vi "Structure Handler.vi"() -> ()   [LabVIEW 2010] (continued)
            n13 = call-poly <vilib>:"DB Tools Open Connection.vi"("connection information"=w16) -> ("error out"=w19:errorcluster, "connection reference"=w26:T17)  [unwired: 7 in]
            n14 = call-poly <vilib>:"DB Tools Execute Query.vi"("error in (no error)"=w19, "SQL query"="SELECT Structure_Summary.Structure_ID, Structure_Summary.Structure_Name, Structure_Summary.Num_Atoms, DFT_Summary.Folder, DFT_Summary.Parent_Folder, DFT_Summary.[Calculation_Time_(Hrs)], OSZICAR_Summary.[Final_Energy_(eV)]\nFROM (DFT_Summary RIGHT JOIN Structure_Summary ON DFT_Summary.CONTCAR_Structure_ID = Structure_Summary.Structure_ID) LEFT JOIN OSZICAR_Summary ON DFT_Summary.OSZICAR_ID = OSZICAR_Summary.OSZICAR_ID\nORDER BY  DFT_Summary.Parent_Folder, Structure_Summary.Structure_Name;", "connection reference"=w26) -> ("error out"=w21:errorcluster, "recordset reference"=w23:T18)  [unwired: 5 in]
            n15 = call "Column Headers from SQL Query Recordset.vi"("error in (no error)"=w21, "recordset reference"=w23) -> ("error out"=w20:errorcluster, "columns"=w14:string[], "Recordset reference Out"=w22:T18)  [unwired: 6 in, 1 out]
            n16 = call-poly <vilib>:"DB Tools Fetch Recordset Data.vi"("error in (no error)"=w20, "recordset reference"=w22) -> ("error out"=w24:errorcluster, "recordset data"=w18:variant[][], "recordset reference out"=w25:T18)  [unwired: 3 in]
            n17 = for {
              tunnel: w18 -> [w30] mode=indexing
              tunnel: [w29] -> w17 mode=indexing
              n18 = for {
                tunnel: w30 -> [w33] mode=indexing
                tunnel: [w31] -> w29 mode=indexing
                n19 = xnode "Database Variant To Data"("database variant"=w33, "type"="") -> ("data"=w31:string)  [unwired: 1 in, 1 out]
              }
            }
            n20 = call-poly <vilib>:"DB Tools Free Object.vi"("error in (no error)"=w24, "recordset reference"=w25) -> ("error out"=w28:errorcluster, "connection reference"=w27:T17)  [unwired: 8 in]
            n21 = call <vilib>:"DB Tools Close Connection.vi"("error in (no error)"=w28, "connection reference"=w27) -> ()  [unwired: 5 in, 1 out]
            n22 = property on="2nd search column name" class="CmbBox"("Strings[]"=w14) -> ()  [unwired: 2 in, 2 out]
            n23 = property on="Database Entries" class="MCListbox (strict)"("ColHdrString"=w14, "ItemNames"=w17) -> ()  [unwired: 2 in, 2 out]
            n24 = property on="1st search column name" class="CmbBox"("Strings[]"=w14) -> ()  [unwired: 2 in, 2 out]
          }
          frame Default {
          }
          frame "VASP" {
            n25 = property on="INCAR Defaults" class="LstBox (strict)"("Val(Sgnl)"=0 ("Value (Signaling)")) -> (error out=w66:errorcluster)  [unwired: 2 in, 1 out]
            n26 = property on="K-Points Tab" class="TabCtl (strict)"(error in=w66, "Val(Sgnl)"=enum32{"Automatic", "Manual"}."Automatic" ("K-Points Tab")) -> ()  [unwired: 1 in, 2 out]
          }
        }
      }
      event "Input Structure File": Value Change {
        n27 = event-data() -> ()  [unwired: 1 in, 5 out]
        n28 = call <vilib>:"Get File Extension.vi"("file"="Input Structure File") -> ("lowercase file extension"=w83:string)  [unwired: 7 in, 3 out]
        n29 = Strip Path(path="Input Structure File") -> (stripped path=w80:path)  [unwired: 1 out]
        n30 = case shown="\"out\"" w83 {
          tunnel: "Input Structure File" -> [w93 w95 w97 _]
          tunnel: [w92 w94 w96 _] -> w75
          frame "CONTCAR", "POSCAR", Default {
            n31 = call "Parse POSCAR.vi"("POSCAR File"=w93) -> ("Structure"=w92:T3)  [unwired: 7 in, 3 out]
          }
          frame "cif" {
            n32 = call "Parse CIF File from ATK.vi"("CIF File from ATK"=w95) -> ("Atomic Structure"=w94:T3)  [unwired: 10 in]
          }
          frame "out" {
            n33 = call "Parse GULP Output file.vi"("GULP output file"=w97) -> ("Final Structure"=w96:T3)  [unwired: 5 in, 5 out]
          }
          frame ".gin" {
          }
        }
        n34 = Strip Path(path=w80) -> (name=w86:string)  [unwired: 1 out]
        n35 = Build Path(base path=w80, name or relative path="README.txt") -> (appended path=w82:path)
        n36 = local write "Structure Name"(w86) -> ()
        n37 = call <vilib>:"Trim Whitespace.vi"("string"=w86) -> ("trimmed string"=w85:string)  [unwired: 1 in]
        n38 = call <vilib>:"Check if File or Folder Exists.vi"("path"=w82) -> ("file or folder exists?"=w81:bool)  [unwired: 8 in, 2 out]
        n39 = local write "VASPIFY Folder Name"(w85) -> ()
        n40 = Unbundle By Name(w75) -> ("Lattice vector c"=w78:dbl[])
        n41 = case shown="True" w81 {
          tunnel: w82 -> [_ w91]
          tunnel: [_ w88] -> w73
          tunnel: [_ w87] -> w72
          frame False {
          }
          frame True {
            n42 = call-poly <vilib>:"Read From Spreadsheet File.vi"("file path (dialog if empty)"=w91) -> ("all rows"=w90:string[][])  [unwired: 6 in, 4 out]
            n43 = Index Array(array=w90, index (col) #1=0 ("disabled index (col)")) -> (element #1=w88:string[], element #2=w87:string[])  [unwired: 3 in]
          }
        }
        n44 = call-poly <vilib>:"Vector Norm.vi"("Input Vector"=w78) -> ("norm"=w77:dbl)  [unwired: 9 in, 1 out]
        n45 = property on="Crop Range" class="Slide (strict)"("Scale.Maximum"=w77) -> ()  [unwired: 2 in, 2 out]
        n46 = Build Array(w75) -> (w76:T1)
        n47 = local write "Last Structures"(w76) -> ()
        n48 = property on="Current Atomic Structure" class="Clust (strict)"("Val(Sgnl)"=w75) -> ()  [unwired: 2 in, 2 out]
        n49 = local write "Headers"(w73) -> ()
        n50 = local write "Values"(w72) -> ()
        n51 = Build Array(w73, w72) -> (w70:string[][])
        n52 = Transpose 2D Array(2D array=w70) -> (transposed array=w69:string[][])
        n53 = Array To Spreadsheet String(array=w69, 3:"%s" ("format string")) -> (spreadsheet string=w74:string)  [unwired: 1 in]
        n54 = local write "Title"(w74) -> ()
      }
      event "Undo Last": Value Change {
        n55 = event-data() -> ()  [unwired: 1 in, 5 out]
        n56 = local read "Last Structures"() -> (w99:T1)
        n57 = Array Size(array=w99) -> (size(s)=w98:i32)
        n58 = case shown="1" w98 {
          tunnel: [w105 w108] -> w101
          tunnel: [w104 w107] -> w100
          tunnel: w99 -> [w104 w106]
          frame 1 {
            n59 = Index Array(array=w104) -> (element=w105:T3)  [unwired: 1 in]
          }
          frame Default {
            n60 = Delete From Array(array=w106, index=0) -> (deleted portion=w108:T3, array with subset deleted=w107:T1)  [unwired: 1 in]
          }
        }
        n61 = Unbundle By Name(w101) -> ("Lattice vector c"=w103:dbl[])
        n62 = local write "Last Structures"(w100) -> ()
        n63 = property on="Current Atomic Structure" class="Clust (strict)"("Val(Sgnl)"=w101) -> ()  [unwired: 2 in, 2 out]
        n64 = call-poly <vilib>:"Vector Norm.vi"("Input Vector"=w103) -> ("norm"=w102:dbl)  [unwired: 9 in, 1 out]
        n65 = property on="Crop Range" class="Slide (strict)"("Scale.Maximum"=w102) -> ()  [unwired: 2 in, 2 out]
      }
      event "Database Entries": Value Change {
        n66 = event-data() -> ()  [unwired: 1 in, 5 out]
        n67 = case shown="Default" "Database Entries" {
          selector: "Database Entries" -> [_ w124]
          frame -1 {
          }
          frame Default {
            n68 = local read "Database UDL"() -> (w123:path)
            n69 = property on="Database Entries" class="MCListbox (strict)"() -> ("ItemNames"=w130:string[][])  [unwired: 2 in, 2 out]
            n70 = Index Array(array=w130, index (row)=w124, index (col)=0 ("disabled index (col)")) -> (element=w121:string)
            n71 = property on="Current Atomic Structure" class="Clust (strict)"("Val(Sgnl)"=w112) -> ()  [unwired: 2 in, 2 out]
            n72 = Unbundle By Name(w112) -> ("Structure Name"=w125:string, "Lattice vector c"=w128:dbl[])
            n73 = local write "Structure Name"(w125) -> ()
            n74 = call <vilib>:"Trim Whitespace.vi"("string"=w125) -> ("trimmed string"=w126:string)  [unwired: 1 in]
            n75 = call-poly <vilib>:"Vector Norm.vi"("Input Vector"=w128) -> ("norm"=w127:dbl)  [unwired: 9 in, 1 out]
            n76 = flat-sequence {
              tunnel: w123 -> [w133]
              tunnel: [w132] -> w122
              tunnel: [w131] -> w119
              tunnel: [w138] -> w112
              tunnel: w122 -> [w137]
              tunnel: w121 -> [w136]
              tunnel: [w135] -> w120
              tunnel: [w134] -> w118
              tunnel: [w140] -> _
              tunnel: w120 -> [w140]
              tunnel: [w139] -> w117
              tunnel: [w141] -> w113
              frame #0 {
                n77 = call-poly <vilib>:"DB Tools Open Connection.vi"("connection information"=w133) -> ("connection reference"=w132:T17)  [unwired: 7 in, 1 out]
                n78 = Tick Count (ms)() -> (millisecond timer value=w131:u32)
              }
              frame #1 {
                n79 = call "Import Structure from DB.vi"("Structure ID"=w136, "connection reference"=w137) -> ("Loaded Structure"=w138:T3, "connection reference out"=w135:T17)  [unwired: 7 in, 1 out]
                n80 = Tick Count (ms)() -> (millisecond timer value=w134:u32)
              }
              frame #2 {
                n81 = Tick Count (ms)() -> (millisecond timer value=w139:u32)
                n82 = call <vilib>:"DB Tools Close Connection.vi"("connection reference"=w140) -> ()  [unwired: 6 in, 1 out]
              }
              frame #3 {
                n83 = Tick Count (ms)() -> (millisecond timer value=w141:u32)
              }
            }
            n84 = Tick Count (ms)() -> (millisecond timer value=w116:u32)
            n85 = local write "VASPIFY Folder Name"(w126) -> ()
            n86 = property on="Crop Range" class="Slide (strict)"("Scale.Maximum"=w127) -> ()  [unwired: 2 in, 2 out]
            n87 = Build Array(w112) -> (w111:T1)
            n88 = local write "Last Structures"(w111) -> ()
            n89 = Build Array(w119, w118, w117, w113) -> (w115:u32[])
            n90 = Subtract(x=w115, y=w116) -> (x-y=→"x-y":u32[])
          }
        }
      }
      event "Apply Filter": Value Change {
        n91 = event-data() -> ()  [unwired: 1 in, 5 out]
        n92 = local read "Database UDL"() -> (w148:path)
        n93 = call "Query Builder - Dynamic Columns.vi"("Date-Time Column Name"="DFT_Summary.[LinuxIFC_Date]", "Query Build Cluster"="Query Filter") -> ("Where Statement"=w145:string)  [unwired: 9 in]
        n94 = call-poly <vilib>:"DB Tools Open Connection.vi"("connection information"=w148) -> ("error out"=w151:errorcluster, "connection reference"=w158:T17)  [unwired: 7 in]
        n95 = Concatenate Strings("SELECT Structure_Summary.Structure_ID, Structure_Summary.Structure_Name, Structure_Summary.Num_Atoms, DFT_Summary.Folder, DFT_Summary.Parent_Folder, DFT_Summary.[Calculation_Time_(Hrs)], OSZICAR_Summary.[Final_Energy_(eV)]\nFROM (DFT_Summary RIGHT JOIN Structure_Summary ON DFT_Summary.CONTCAR_Structure_ID = Structure_Summary.Structure_ID) LEFT JOIN OSZICAR_Summary ON DFT_Summary.OSZICAR_ID = OSZICAR_Summary.OSZICAR_ID\n" ("SQL query"), w145, " ORDER BY  DFT_Summary.Parent_Folder, Structure_Summary.Structure_Name;") -> (w142:string)
        n96 = call-poly <vilib>:"DB Tools Execute Query.vi"("error in (no error)"=w151, "SQL query"=w142, "connection reference"=w158) -> ("error out"=w153:errorcluster, "recordset reference"=w155:T18)  [unwired: 5 in]
        n97 = call "Column Headers from SQL Query Recordset.vi"("error in (no error)"=w153, "recordset reference"=w155) -> ("error out"=w152:errorcluster, "columns"=w147:string[], "Recordset reference Out"=w154:T18)  [unwired: 6 in, 1 out]
        n98 = property on="1st search column name" class="CmbBox"("Strings[]"=w147) -> ()  [unwired: 2 in, 2 out]
        n99 = call-poly <vilib>:"DB Tools Fetch Recordset Data.vi"("error in (no error)"=w152, "recordset reference"=w154) -> ("error out"=w156:errorcluster, "recordset data"=w150:variant[][], "recordset reference out"=w157:T18)  [unwired: 3 in]
        n100 = for {
          tunnel: w150 -> [w163] mode=indexing
          tunnel: [w162] -> w149 mode=indexing
          n101 = for {
            tunnel: w163 -> [w166] mode=indexing
            tunnel: [w164] -> w162 mode=indexing
            n102 = xnode "Database Variant To Data"("database variant"=w166, "type"="") -> ("data"=w164:string)  [unwired: 1 in, 1 out]
          }
        }
        n103 = call-poly <vilib>:"DB Tools Free Object.vi"("error in (no error)"=w156, "recordset reference"=w157) -> ("error out"=w160:errorcluster, "connection reference"=w159:T17)  [unwired: 8 in]
        n104 = call <vilib>:"DB Tools Close Connection.vi"("error in (no error)"=w160, "connection reference"=w159) -> ()  [unwired: 5 in, 1 out]
        n105 = property on="Database Entries" class="MCListbox (strict)"("ColHdrString"=w147, "ItemNames"=w149) -> ()  [unwired: 2 in, 2 out]
      }
      event "Scale", "Current Atomic Structure", "Options": Value Change {
        # "\"Base\" Object is the top level object\nAll atoms are sub-objects of Base"
        n106 = event-data() -> ()  [unwired: 1 in, 5 out]
        n107 = local read "Base Object"() -> (w202:refnum<vi>)
        n108 = Close Reference(reference=w202) -> (error out=w201:errorcluster)  [unwired: 1 in]
        n109 = call <vilib>:"Create Object.vi"("error in (no error)"=w201, "Name"="Base") -> ("Scene:New Object"=w212:refnum<vi>)  [unwired: 9 out]
        n110 = call "Create Structure ID from Structure.vi"("Structure"="Current Atomic Structure") -> ("Structure ID"=w200:string)  [unwired: 10 in]
        "Structure ID" <- w200
        n111 = call "Render Structure.vi"("Options"="Options", "Atom Size"="Atom Size", "Scale"="Scale", "Atomic Structure"="Current Atomic Structure", "Base Object"=w212) -> ("Object with atoms"=→"Scene Display" →"Base Object":refnum<vi>)  [unwired: 6 in]
        n112 = property on="Structure ID" class="Str"("Val(Sgnl)"=w200) -> ()  [unwired: 2 in, 2 out]
        n113 = case shown="True" "Auto-Setup Camera" {
          tunnel: "Current Atomic Structure" -> [_ w234]
          frame False {
          }
          frame True {
            n114 = local read "Scale"() -> (w233:dbl)
            n115 = Unbundle By Name(w234) -> ("Lattice vector a"=w240:dbl[], "Lattice vector b"=w241:dbl[], "Lattice vector c"=w235:dbl[])
            n116 = Negate(x=w240) -> (-x=w242:dbl[])
            n117 = Array To Cluster(array=w241) -> (cluster=w230:T19)
            n118 = Compound Arithmetic op=ADD(w240, w241, w235) -> (w237:dbl[])
            n119 = Multiply(x=w242, y=2.0 ("Numeric")) -> (x*y=w244:dbl[])
            n120 = Divide(x=w237, y=2.0) -> (x/y=w238:dbl[])
            n121 = Array To Cluster(array=w244) -> (cluster=w232:cluster{"[0]":dbl, "[1]":dbl, "[2]":dbl})
            n122 = Multiply(x=w238, y=w233) -> (x*y=w239:dbl[])
            n123 = Array To Cluster(array=w239) -> (cluster=w231:cluster{"[0]":dbl, "[1]":dbl, "[2]":dbl})
            n124 = invoke on="Scene Display" class="SceneGraphDisp (strict)" method="Setup Camera"("Camera Position"=w232, "Target"=w231, "Up Direction"=w230) -> ()  [unwired: 3 in, 6 out]
          }
        }
        n125 = Wait (ms)(milliseconds to wait=u32 1) -> ()  [unwired: 1 out]
        n126 = Unbundle By Name("Current Atomic Structure") -> ("Atoms Array"=w208:T20)
        n127 = for {
          tunnel: w208 -> [w219] mode=indexing
          shift-right: [w215] -> w207
          shift-left: string[][] [] -> [w214]
          n128 = Unbundle By Name(w219) -> ("Atom Name"=w216:string, "Positions (Direct)"=w218:dbl[][], "Positions (Cartesian)"=w217:dbl[][])
          n129 = for {
            tunnel: w218 -> [w229] mode=indexing
            tunnel: w217 -> [w228] mode=indexing
            tunnel: w216 -> [w227]
            shift-right: [w223] -> w215
            shift-left: w214 -> [w222]
            i -> [w221]
            n130 = Number To Decimal String(number=w221) -> (decimal integer string=w220:string)  [unwired: 1 in]
            n131 = Number To Fractional String(number=w229) -> (F-format string=w226:string[])  [unwired: 3 in]
            n132 = Number To Fractional String(number=w228) -> (F-format string=w225:string[])  [unwired: 3 in]
            n133 = Build Array (concatenate)(w227, w226, w225, w220) -> (w224:string[])
            n134 = Build Array (concatenate)(w222, w224) -> (w223:string[][])
          }
        }
        n135 = property on="Atom List" class="MCListbox (strict)"("ItemNames"=w207) -> ()  [unwired: 2 in, 2 out]
      }
      event "Add Bulk": Value Change {
        n136 = event-data() -> ()  [unwired: 1 in, 5 out]
        n137 = local read "Bulk Options"() -> (w247:T1)
        n138 = local read "Current Atomic Structure"() -> (w250:T3)
        n139 = Build Array (concatenate)(w247, "Base 111 Structures") -> (w245:T1)
        n140 = Index Array(array=w245, index="Padding Options") -> (element=w251:T3)
        n141 = case shown="\"Pad on Left\", Default" "Where to pad?" {
          tunnel: w251 -> [w255 w260]
          tunnel: w250 -> [w256 w259]
          tunnel: [w253 w257] -> w249
          frame "Pad on Left", Default {
            n142 = Unbundle By Name(w255) -> ("Lattice vector c"=w254:dbl[])
            n143 = call "Merge Two Structures (Cuboid).vi"("Translation Vector (1 to 2)"=w254, "Atomic Structure 2"=w256, "Atomic Structure 1"=w255) -> ("Atomic Structure of 1 + 2 by T"=w253:T3)  [unwired: 8 in]
          }
          frame "Pad on Right" {
            n144 = Unbundle By Name(w259) -> ("Lattice vector c"=w258:dbl[])
            n145 = call "Merge Two Structures (Cuboid).vi"("Translation Vector (1 to 2)"=w258, "Atomic Structure 2"=w260, "Atomic Structure 1"=w259) -> ("Atomic Structure of 1 + 2 by T"=w257:T3)  [unwired: 8 in]
          }
        }
        n146 = property on="Current Atomic Structure" class="Clust (strict)"("Val(Sgnl)"=w249) -> ()  [unwired: 2 in, 2 out]
      }
      event "Crop Range": Value Change {
        n147 = event-data() -> ()  [unwired: 1 in, 5 out]
        n148 = local read "Last Structures"() -> (w262:T1)
        n149 = Unbundle("Crop Range") -> (w267:dbl, w266:dbl)
        n150 = Max & Min(x=w267, y=w266) -> (max(x,y)=w265:dbl, min(x,y)=w264:dbl)
        n151 = Index Array(array=w262) -> (element=w261:T3)  [unwired: 1 in]
        n152 = call "Crop Structure.vi"("Cropping Index"="Cropping Index", "Upper Bound Z"=w265, "Lower bound Z"=w264, "Input Structure"=w261) -> ("Cropped Structure"=w269:T3)  [unwired: 7 in]
        n153 = property on="Current Atomic Structure" class="Clust (strict)"("Val(Sgnl)"=w269) -> ()  [unwired: 2 in, 2 out]
      }
      event "Prickle Distance (A)": Value Change {
        n154 = event-data() -> ()  [unwired: 1 in, 5 out]
        n155 = local read "Last Structures"() -> (w271:T1)
        n156 = Index Array(array=w271) -> (element=w270:T3)  [unwired: 1 in]
        n157 = call "Prickle a structure towards its boundary.vi"("Prickle Distance (Cartesian)"="Prickle Distance (A)", "Input Structure"=w270) -> ("Prickled Structure"=w272:T3)  [unwired: 9 in]
        n158 = property on="Current Atomic Structure" class="Clust (strict)"("Val(Sgnl)"=w272) -> ()  [unwired: 2 in, 2 out]
      }
      event "Translation Vector (Cartesian)": Value Change {
        n159 = event-data() -> ()  [unwired: 1 in, 5 out]
        n160 = local read "Last Structures"() -> (w275:T1)
        n161 = Index Array(array=w275) -> (element=w274:T3)  [unwired: 1 in]
        n162 = call "Translate Structure.vi"("Translation Vector (Cartesian)"="Translation Vector (Cartesian)", "Atomic Structure"=w274) -> ("Shifted Structure"=w276:T3)  [unwired: 9 in]
        n163 = property on="Current Atomic Structure" class="Clust (strict)"("Val(Sgnl)"=w276) -> ()  [unwired: 2 in, 2 out]
      }
      event "Suggest Supercell Draw Box": Value Change {
        w293 = 0.0 ("norm")
        n164 = event-data() -> ()  [unwired: 1 in, 5 out]
        n165 = local read "Last Structures"() -> (w279:T1)
        n166 = Index Array(array=w279) -> (element=w278:T3)  [unwired: 1 in]
        n167 = Unbundle By Name(w278) -> ("Lattice vector a"=w298:dbl[], "Lattice vector b"=w297:dbl[], "Lattice vector c"=w292:dbl[])
        n168 = call-poly <vilib>:"Vector Norm.vi"("Input Vector"=w298) -> ("norm"=w296:dbl)  [unwired: 9 in, 1 out]
        n169 = call-poly <vilib>:"Vector Norm.vi"("Input Vector"=w297) -> ("norm"=w295:dbl)  [unwired: 9 in, 1 out]
        n170 = call-poly <vilib>:"Vector Norm.vi"("Input Vector"=w292) -> ("norm"=w294:dbl)  [unwired: 9 in, 1 out]
        n171 = Bundle("norm"=w293, "norm"=w296, "norm"=w293, "norm"=w295, "norm"=w293, "norm"=w294) -> (w291:T21)  [unwired: 1 in]
        n172 = Multiply(x=w291, y=1.0 ("norm")) -> (x*y=w289:T21)
        n173 = Unbundle(w289) -> ("norm"=w288:dbl, "norm"=w287:dbl, "norm"=w286:dbl, "norm"=w285:dbl, "norm"=w284:dbl, "norm"=w283:dbl)
        n174 = Bundle("norm"=w288, "norm"=w287) -> (w282:cluster{"norm":dbl, "norm":dbl})  [unwired: 1 in]
        n175 = Bundle("norm"=w286, "norm"=w285) -> (w281:cluster{"norm":dbl, "norm":dbl})  [unwired: 1 in]
        n176 = Bundle("norm"=w284, "norm"=w283) -> (w280:cluster{"norm":dbl, "norm":dbl})  [unwired: 1 in]
        n177 = local write "Supercell Draw Box Y"(w281) -> ()
        n178 = local write "Supercell Draw Box X"(w282) -> ()
        n179 = local write "Supercell Draw Box Z"(w280) -> ()
        n180 = property on="Supercell Draw Box Z" class="Slide (strict)"("Val(Sgnl)"=w280) -> ()  [unwired: 2 in, 2 out]
      }
      event "Supercell Draw Box Z", "Supercell Draw Box Y", "Supercell Draw Box X": Value Change {
        n181 = event-data() -> ()  [unwired: 1 in, 5 out]
        n182 = Unbundle("Supercell Draw Box X") -> (w309:dbl, w308:dbl)
        n183 = Unbundle("Supercell Draw Box Y") -> (w307:dbl, w306:dbl)
        n184 = Unbundle("Supercell Draw Box Z") -> (w305:dbl, w304:dbl)
        n185 = Bundle(w309, w308, w307, w306, w305, w304) -> (w313:cluster{dbl, dbl, dbl, dbl, dbl, dbl})  [unwired: 1 in]
        n186 = local read "Last Structures"() -> (w301:T1)
        n187 = Index Array(array=w301) -> (element=w300:T3)  [unwired: 1 in]
        n188 = call "Supercell Structure into a Box.vi"("Keep old lattice vectors?"=FALSE, "Draw Box"=w313, "Subcrystal"=w300) -> ("error out"=w299:errorcluster, "Expanded cubic Structure"=w303:T3)  [unwired: 6 in, 1 out]
        n189 = call <vilib>:"Clear Errors.vi"("error in (no error)"=w299) -> ()  [unwired: 6 in, 1 out]
        n190 = property on="Current Atomic Structure" class="Clust (strict)"("Val(Sgnl)"=w303) -> ()  [unwired: 2 in, 2 out]
      }
      event Value Change {
        n191 = event-data() -> ()  [unwired: 1 in, 5 out]
        n192 = local read "Last Structures"() -> (w315:T1)
        n193 = Index Array(array=w315) -> (element=w314:T3)  [unwired: 1 in]
        n194 = call "Matrix Transform Structure.vi"("Matrix Transform"="Matrix Transform", "Original Structure"=w314) -> ("After Transform"=w316:T3)  [unwired: 9 in]
        n195 = property on="Current Atomic Structure" class="Clust (strict)"("Val(Sgnl)"=w316) -> ()  [unwired: 2 in, 2 out]
      }
      event "New a Axis", "New b Axis", "New c Axis": Value Change {
        w329 = -0.01 ("norm")
        n196 = event-data() -> ()  [unwired: 1 in, 5 out]
        n197 = case shown="False" "Lock c" {
          tunnel: "New c Axis" -> [w365 w391]
          tunnel: "Lock a" -> [w366 w392]
          tunnel: [w364 w390] -> w336
          tunnel: [w363 w389] -> w334
          tunnel: [w362 w388] -> w335
          tunnel: "New a Axis" -> [w361 w387]
          tunnel: "Lock b" -> [w360 w386]
          tunnel: "New b Axis" -> [w359 w385]
          frame True {
            n198 = case shown="False" w366 {
              tunnel: w365 -> [w368 w376]
              tunnel: [w370 w377] -> w364
              tunnel: [w367 w372] -> w362
              tunnel: [w368 w371] -> w363
              tunnel: w361 -> [w367 w375]
              tunnel: w360 -> [_ w374]
              tunnel: w359 -> [_ w373]
              frame True {
                n199 = call <vilib>:"Cross Product.vi"("B Vector"=w368, "A Vector"=w367) -> ("Cross Product"=w370:dbl[])  [unwired: 8 in, 1 out]
                n200 = local write "Lock b"(FALSE ("Lock b")) -> ()
                n201 = local write "New b Axis"(w370) -> ()
              }
              frame False {
                n202 = case shown="False" w374 {
                  tunnel: [w380 w382] -> w377
                  tunnel: w376 -> [w378 w384]
                  tunnel: w375 -> [_ _]
                  tunnel: w373 -> [w380 _]
                  tunnel: [w379 w383] -> w372
                  tunnel: [w378 w384] -> w371
                  frame True {
                    n203 = call <vilib>:"Cross Product.vi"("B Vector"=w378, "A Vector"=w380) -> ("Cross Product"=w379:dbl[])  [unwired: 8 in, 1 out]
                    n204 = local write "Lock a"(FALSE ("Lock b")) -> ()
                    n205 = local write "New a Axis"(w379) -> ()
                  }
                  frame False {
                    w383 = dbl[] [1.0, 0.0, 0.0] ("A Vector")
                    n206 = local write "New a Axis"(w383) -> ()
                    n207 = call <vilib>:"Cross Product.vi"("B Vector"=w384, "A Vector"=w383) -> ("Cross Product"=w382:dbl[])  [unwired: 8 in, 1 out]
                    n208 = local write "New b Axis"(w382) -> ()
                  }
                }
              }
            }
          }
          frame False {
            n209 = case shown="False" w392 {
              tunnel: w391 -> [w394 w402]
              tunnel: [w396 w403] -> w390
              tunnel: [w393 w398] -> w388
              tunnel: [w394 w397] -> w389
              tunnel: w387 -> [w393 w401]
              tunnel: w386 -> [_ w400]
              tunnel: w385 -> [_ w399]
              frame True {
                n210 = call <vilib>:"Cross Product.vi"("B Vector"=w394, "A Vector"=w393) -> ("Cross Product"=w396:dbl[])  [unwired: 8 in, 1 out]
                n211 = local write "Lock b"(FALSE ("Lock b")) -> ()
                n212 = local write "New b Axis"(w396) -> ()
              }
              frame False {
                n213 = case shown="False" w400 {
                  tunnel: [w406 w408] -> w403
                  tunnel: w402 -> [w404 w410]
                  tunnel: w401 -> [_ _]
                  tunnel: w399 -> [w406 _]
                  tunnel: [w405 w409] -> w398
                  tunnel: [w404 w410] -> w397
                  frame True {
                    n214 = call <vilib>:"Cross Product.vi"("B Vector"=w404, "A Vector"=w406) -> ("Cross Product"=w405:dbl[])  [unwired: 8 in, 1 out]
                    n215 = local write "Lock a"(FALSE ("Lock b")) -> ()
                    n216 = local write "New a Axis"(w405) -> ()
                  }
                  frame False {
                    w409 = dbl[] [1.0, 0.0, 0.0] ("A Vector")
                    n217 = local write "New a Axis"(w409) -> ()
                    n218 = call <vilib>:"Cross Product.vi"("B Vector"=w410, "A Vector"=w409) -> ("Cross Product"=w408:dbl[])  [unwired: 8 in, 1 out]
                    n219 = local write "New b Axis"(w408) -> ()
                  }
                }
              }
            }
          }
        }
        n220 = local read "Last Structures"() -> (w319:T1)
        n221 = Index Array(array=w319) -> (element=w318:T3)  [unwired: 1 in]
        n222 = disable-structure shown="Enabled" {
          disable-tunnel: w318 -> [w355 w358]
          disable-tunnel: [w354 w358] -> w322
          frame Disabled {
            n223 = call "Find Subcrystal.vi"("Atomic Structure"=w355) -> ("Base Atom Position (Cartesian)"=w356:dbl[], "Subcrystal"=w357:T3)  [unwired: 8 in, 1 out]
            n224 = call "Translate Structure.vi"("Translation Vector (Cartesian)"=w356, "Atomic Structure"=w357) -> ("Shifted Structure"=w354:T3)  [unwired: 9 in]
          }
          frame Enabled {
          }
        }
        n225 = Unbundle By Name(w318) -> ("Lattice vector a"=w325:dbl[], "Lattice vector b"=w324:dbl[], "Lattice vector c"=w323:dbl[])
        n226 = call-poly <vilib>:"Vector Norm.vi"("Input Vector"=w335) -> ("norm"=w346:dbl)  [unwired: 9 in, 1 out]
        n227 = call-poly <vilib>:"Vector Norm.vi"("Input Vector"=w336) -> ("norm"=w344:dbl)  [unwired: 9 in, 1 out]
        n228 = call-poly <vilib>:"Vector Norm.vi"("Input Vector"=w334) -> ("norm"=w343:dbl)  [unwired: 9 in, 1 out]
        n229 = Divide(x=w335, y=w346) -> (x/y=w342:dbl[])
        n230 = Divide(x=w336, y=w344) -> (x/y=w341:dbl[])
        n231 = Divide(x=w334, y=w343) -> (x/y=w340:dbl[])
        n232 = call-poly <vilib>:"Vector Norm.vi"("Input Vector"=w325) -> ("norm"=w332:dbl)  [unwired: 9 in, 1 out]
        n233 = call-poly <vilib>:"Vector Norm.vi"("Input Vector"=w324) -> ("norm"=w331:dbl)  [unwired: 9 in, 1 out]
        n234 = call-poly <vilib>:"Vector Norm.vi"("Input Vector"=w323) -> ("norm"=w330:dbl)  [unwired: 9 in, 1 out]
        n235 = Build Array(w342, w341, w340) -> (w333:T9)
        n236 = local write "Matrix Transform"(w333) -> ()
        n237 = call "Matrix Transform Structure.vi"("Matrix Transform"=w333, "Original Structure"=w322) -> ("After Transform"=w321:T3)  [unwired: 9 in]
        n238 = Bundle("norm"=w329, "norm"=w332, "norm"=w329, "norm"=w331, "norm"=w329, "norm"=w330) -> (w328:T21)  [unwired: 1 in]
        n239 = Multiply(x=w328, y=1.01 ("norm")) -> (x*y=w327:T21)
        n240 = disable-structure shown="Enabled" {
          disable-tunnel: w327 -> [w352 _]
          disable-tunnel: w321 -> [w351 w353]
          disable-tunnel: [w350 w353] -> w320
          frame Disabled {
            n241 = call "Supercell Structure into a Box.vi"("Center Subcrystal"=TRUE, "Draw Box"=w352, "Subcrystal"=w351) -> ("Expanded cubic Structure"=w350:T3)  [unwired: 6 in, 2 out]
          }
          frame Enabled {
          }
        }
        n242 = property on="Current Atomic Structure" class="Clust (strict)"("Val(Sgnl)"=w320) -> ()  [unwired: 2 in, 2 out]
      }
      event "Accept These Changes": Value Change {
        n243 = event-data() -> ()  [unwired: 1 in, 5 out]
        n244 = local read "Current Atomic Structure"() -> (w411:T3)
        n245 = local read "Last Structures"() -> (w413:T1)
        n246 = Unbundle By Name(w411) -> ("Lattice vector c"=w419:dbl[])
        n247 = Array Size(array=w413) -> (size(s)=w414:i32)
        n248 = Index Array(array=w419, index=2) -> (element=w417:dbl)
        n249 = Bundle("element"=0.0, "Numeric"=w417) -> (w415:cluster{"element":dbl, "Numeric":dbl})  [unwired: 1 in]
        n250 = local write "Crop Range"(w415) -> ()
        n251 = case shown="5" w414 {
          tunnel: w413 -> [w425 w426]
          tunnel: w411 -> [w422 w427]
          tunnel: [w421 w428] -> w412
          frame 5 {
            n252 = Rotate 1D Array(1:w425, 2:1 ("n")) -> (0:w424:T1)
            n253 = Replace Array Subset(array=w424, new element=w422, index=0) -> (w421:T1)
          }
          frame Default {
            n254 = Build Array (concatenate)(w427, w426) -> (w428:T1)
          }
        }
        "Last Structures" <- w412
      }
      event "Rotation": Value Change {
        n255 = event-data() -> ()  [unwired: 1 in, 5 out]
        n256 = call "Make Rotation Matrix.vi"("Rotation Axis"="Rotation Axis", "Rotation Angle (Degree)"="Rotation") -> ("Rotation Matrix"=w429:T9)  [unwired: 9 in]
        n257 = local read "Base Object"() -> (w431:refnum<vi>)
        n258 = for {
          tunnel: w429 -> [w449] mode=indexing
          tunnel: [w448] -> w437 mode=indexing
          n259 = for {
            tunnel: [w450] -> w448 mode=indexing
            tunnel: w449 -> [w450] mode=indexing
          }
        }
        n260 = Array To Cluster(array="Rotation Axis") -> (cluster=w441:T22)
        n261 = call <vilib>:"Clear Transformation.vi"("Object Refnum In"=w431) -> ("Object Refnum Out"=w430:refnum<vi>)  [unwired: 9 in, 1 out]
        n262 = disable-structure shown="Disabled" {
          disable-tunnel: "Rotation" -> [w446 _]
          disable-tunnel: w441 -> [w445 _]
          disable-tunnel: [w444 w447] -> w432
          disable-tunnel: w430 -> [w443 w447]
          frame Disabled {
            n263 = call <vilib>:"Rotate Object.vi"("Angle"=w446, "Axis"=w445, "Scene.Object In"=w443) -> ("Scene.Object Out"=w444:refnum<vi>)  [unwired: 7 in, 1 out]
          }
          frame Enabled {
          }
        }
        n264 = property on="Scene Display" class="SceneGraphDisp (strict)"() -> ("ModelView Matrix"=w439:sgl[][])  [unwired: 2 in, 2 out]
        n265 = Transpose 2D Array(2D array=w437) -> (transposed array=w436:dbl[][])
        n266 = local write "Scene Display"(w432) -> ()
        n267 = local write "Matrix Transform"(w429) -> ()
        n268 = Index Array(array=w439, index (col)=3 ("disabled index (col)")) -> (element=w435:sgl[])  [unwired: 1 in]
        n269 = Build Array (concatenate)(w436, w435) -> (w434:dbl[][])
        n270 = Transpose 2D Array(2D array=w434) -> (transposed array=w433:dbl[][])
        n271 = property on="Scene Display" class="SceneGraphDisp (strict)"("ModelView Matrix"=w433) -> ()  [unwired: 2 in, 2 out]
      }
      event "a lattice factor", "b lattice factor", "c lattice factor": Value Change {
        n272 = event-data() -> ()  [unwired: 1 in, 5 out]
        n273 = local read "Last Structures"() -> (w452:T1)
        n274 = Index Array(array=w452) -> (element=w451:T3)  [unwired: 1 in]
        n275 = call "Structure to Supercell Structure.vi"("c lattice factor"="c lattice factor", "b lattice factor"="b lattice factor", "a lattice factor"="a lattice factor", "Input Structure"=w451) -> ("Supercell Structure"=w456:T3)  [unwired: 7 in]
        n276 = property on="Current Atomic Structure" class="Clust (strict)"("Val(Sgnl)"=w456) -> ()  [unwired: 2 in, 2 out]
      }
      event "K-Points Tab", "Auto Type", "|G| Factor", "Symmetry", "Manual Type", "K-point Mesh", "# Points between": Value Change {
        n277 = event-data() -> ()  [unwired: 1 in, 5 out]
        n278 = local read "Current Atomic Structure"() -> (w458:T3)
        n279 = case shown="\"Automatic\", Default" "K-Points Tab" {
          tunnel: [w466 w467] -> w459
          tunnel: w458 -> [w463 _]
          frame "Automatic", Default {
            n280 = Unbundle By Name(w463) -> ("Lattice vector a"=w462:dbl[], "Lattice vector b"=w461:dbl[], "Lattice vector c"=w460:dbl[])
            n281 = call "Make K-Points File, Auto.vi"("|G| Factor"="|G| Factor", "Lattice vector c"=w460, "Lattice vector b"=w461, "Lattice vector a"=w462, "Auto Type"="Auto Type") -> ("K-Points File"=w466:string)  [unwired: 6 in]
          }
          frame "Manual" {
            n282 = call "Make K-Points File, Manual.vi"("K-point Mesh"="K-point Mesh", "# Points between"="# Points between", "Symmetry"="Symmetry", "Manual Type"="Manual Type") -> ("K-Points File"=w467:string)  [unwired: 7 in]
          }
        }
        "K-Points File" <- w459
      }
      event "VASPify": Value Change {
        n283 = event-data() -> ()  [unwired: 1 in, 5 out]
        n284 = local read "Last Path"() -> (w474:path)
        n285 = call "File Dialog"("start path"=w474) -> ("selected path"=w477:path, "cancelled"=w475:bool, "error out"=w473:errorcluster)  [unwired: 11 in, 1 out]
        "Last Path" <- w477
        n286 = Build Path(base path=w477, name or relative path="VASPIFY Folder Name") -> (appended path=w476:path)
        n287 = case shown="False" w475 {
          tunnel: w476 -> [w479 _]
          tunnel: w473 -> [_ _]
          frame False {
            n288 = Create Folder(path (use dialog)=w479) -> (created path=w478:path)  [unwired: 2 in, 2 out]
            n289 = stacked-sequence {
              tunnel: w478 -> [w480 w484 w488 w494 w524 _ w527]
              frame #0 {
                n290 = local read "POTCAR File"() -> (w481:string)
                n291 = Build Path(base path=w480, name or relative path="POTCAR") -> (appended path=w483:path)
                n292 = Write to Text File(file (use dialog)=w483, text=w481) -> ()  [unwired: 2 in, 3 out]
              }
              frame #1 {
                n293 = local read "INCAR File"() -> (w485:string)
                n294 = Build Path(base path=w484, name or relative path="INCAR") -> (appended path=w487:path)
                n295 = Write to Text File(file (use dialog)=w487, text=w485) -> ()  [unwired: 2 in, 3 out]
              }
              frame #2 {
                n296 = local read "K-Points File"() -> (w489:string)
                n297 = Build Path(base path=w488, name or relative path="KPOINTS") -> (appended path=w491:path)
                n298 = Write to Text File(file (use dialog)=w491, text=w489) -> ()  [unwired: 2 in, 3 out]
              }
              frame #3 {
                n299 = local read "Current Atomic Structure"() -> (w499:T3)
                n300 = case shown="True" "Wiggle one atom by 0.1%" {
                  tunnel: w499 -> [w500 w505]
                  tunnel: [w500 w503] -> w497
                  frame False {
                  }
                  frame True {
                    n301 = Unbundle By Name(w505) -> ("Atoms Array"=w508:T20)
                    n302 = Index Array(array=w508) -> (element=w510:T23)  [unwired: 1 in]
                    n303 = Unbundle By Name(w510) -> ("Positions (Direct)"=w512:dbl[][])
                    n304 = Index Array(array=w512, index (row)=0) -> (element=w502:dbl[])  [unwired: 1 in]
                    n305 = Multiply(x=w502, y=1.0001) -> (x*y=w501:dbl[])
                    n306 = Replace Array Subset(array=w512, new element=w501, index (row)=0) -> (w509:dbl[][])  [unwired: 1 in]
                    n307 = Bundle By Name(cluster=w510, "Positions (Direct)"=w509) -> (w507:T23)
                    n308 = Replace Array Subset(array=w508, new element=w507, index=0) -> (w504:T20)
                    n309 = Bundle By Name(cluster=w505, "Atoms Array"=w504) -> (w503:T3)
                  }
                }
                n310 = Build Path(base path=w494, name or relative path="POSCAR") -> (appended path=w492:path)
                n311 = call "Atoms to POSCAR.vi"("Volume Factor"=1.0, "Atomic Structure"=w497) -> ("POSCAR File"=w495:string)  [unwired: 9 in]
                n312 = Write to Text File(file (use dialog)=w492, text=w495) -> ()  [unwired: 2 in, 3 out]
              }
              frame #4 {
                n313 = local read "Structure Name"() -> (w518:string)
                n314 = call "Write Jobscript for Carbon.vi"("Load VTST for NEB?"="Load VTST for NEB?", "Email?"="Email?", "Expected Walltime"="Expected Walltime", "Nodes and Processors"="Nodes and Processors", "CNM Contract Name"="CNM Contract Name", "Submitname on Carbon"=w518) -> ("Jobscript"=w522:string)  [unwired: 5 in]
                n315 = Build Path(base path=w524, name or relative path="jobscript-") -> (appended path=w521:path)
                n316 = Write to Text File(file (use dialog)=w521, text=w522) -> ()  [unwired: 2 in, 3 out]
              }
              frame #5 {
              }
              frame #6 {
                # "README"
                n317 = Build Array("Headers", "Values") -> (w529:string[][])
                n318 = Build Path(base path=w527, name or relative path="README.txt") -> (appended path=w526:path)
                n319 = Transpose 2D Array(2D array=w529) -> (transposed array=w528:string[][])
                n320 = call-poly <vilib>:"Write To Spreadsheet File.vi"("2D data"=w528, "file path (dialog if empty)"=w526) -> ()  [unwired: 6 in, 1 out]
              }
            }
          }
          frame True {
          }
        }
      }
      event "VASPIFY Folder Name": Value Change {
        n321 = event-data() -> ("NewVal"=w533:string)  [unwired: 1 in, 4 out]
        n322 = call <vilib>:"Trim Whitespace.vi"("string"=w533) -> ("trimmed string"=w532:string)  [unwired: 1 in]
        n323 = local write "VASPIFY Folder Name"(w532) -> ()
      }
      event "GULP": Value Change {
        n324 = event-data() -> ()  [unwired: 1 in, 5 out]
        n325 = local read "Current Atomic Structure"() -> (w543:T3)
        n326 = Unbundle By Name(w543) -> ("Structure Name"=w542:string)
        n327 = call "Atoms to GULP File.vi"("Potentials"="Potentials", "Lattice Vectors"="Lattice Vectors", "Title and Comments"="Title", "Relaxation Type"="Relaxation Type", "Structure"=w543) -> ("GULP File"=w538:string)  [unwired: 6 in]
        n328 = call <vilib>:"Search and Replace Pattern.vi"("string"=w542, "regular expression (\"\")"="[\\s()\\[\\]]" ("regular expression (\"\")"), "replace string (\"\")"="_" ("replace string (\"\")"), "replace all? (F)"=TRUE) -> ("result string"=w541:string)  [unwired: 1 in, 1 out]
        n329 = local read "Last Path"() -> (w549:path)
        n330 = Concatenate Strings(w541, ".gin" ("string")) -> (w539:string)
        n331 = call "GULP Location"("start path"=w549) -> ("selected path"=w548:path, "error out"=w535:errorcluster)  [unwired: 11 in, 2 out]
        n332 = Build Path(base path=w548, name or relative path=w539) -> (appended path=w547:path)
        n333 = case shown="No Error" w535 {
          tunnel: w547 -> [w552 _]
          tunnel: w538 -> [w551 _]
          frame No Error {
            n334 = Write to Text File(file (use dialog)=w552, text=w551) -> ()  [unwired: 2 in, 3 out]
          }
          frame Error {
          }
        }
      }
      event "Save to File": Value Change {
        n335 = event-data() -> ()  [unwired: 1 in, 5 out]
        n336 = local read "Input Structure File"() -> (w555:path)
        n337 = local read "Current Atomic Structure"() -> (w557:T3)
        n338 = call "File Dialog2"("start path"=w555, "default name"="POSCAR") -> ("selected path"=w553:path)  [unwired: 10 in, 3 out]
        n339 = call "Atoms to POSCAR.vi"("Atomic Structure"=w557) -> ("POSCAR File"=w556:string)  [unwired: 10 in]
        n340 = Write to Text File(file (use dialog)=w553, text=w556) -> ()  [unwired: 2 in, 3 out]
      }
      event "INCAR Defaults": Value Change {
        n341 = event-data() -> ()  [unwired: 1 in, 5 out]
        n342 = property on="INCAR Defaults" class="LstBox (strict)"() -> ("Item Names"=w560:string[])  [unwired: 2 in, 2 out]
        n343 = Index Array(array=w560, index="INCAR Defaults") -> (element=w558:string)
        n344 = case shown="\"Dielectric Tensor\"" w558 {
          tunnel: [w562 w572 w573 w574 w575 "#For DOS Calcuations\n# I/O\nICHARG=1\nLWAVE=.FALSE.\nLORBIT=11\nNEDOS=2000  # Number of DOS steps\n\n# Ionic\nIBRION=-1\nISIF=2\nNSW=1\nLREAL=Auto\n\n# Electronic\nISMEAR=-5\nPREC=High\nALGO=Fast\nISPIN=1     # Electron spin, 1=nope, 2=account for spin\nNELM=100\nNELMIN=5\nEDIFF=1E-06  #energy difference to stop relaxation at\n\n# Parallelization\nNPAR=4 # change this to the number of nodes in the job" ("INCAR - Relaxation") "#For Partial Charge Calcuations (PARCHG), you need the WAVECAR file to do this!\n# I/O\nICHARG=1\nLWAVE=.FALSE.\nLORBIT=11\nNEDOS=2000  # Number of DOS n-bands\nLPARD = .TRUE.   # Request PARCHG file if WAVECAR is there.\n\n# Ionic\nIBRION=-1\nISIF=2\nNSW=1\nLREAL=Auto\n\n# Electronic\nISMEAR=-5\nPREC=High\nALGO=Fast\nISPIN=1     # Electron spin, 1=nope, 2=account for spin\nNELM=100\nNELMIN=5\nEDIFF=1E-06  #energy difference to stop relaxation\n\n#Partial Charge\nEINT = 0.0 3 # range of energies to parchg\nLSEPB = 0    # PARCHG by band? True or false\nLSEPK = 0    # PARCHG by k-point? True or false\nIBAND = ?    # Which bands to calculate\nNBMOD = -1   # 0=all bands, -2=partial charge in EINT, -3 Partial chg vs Fermi, >0 IBAND array size\n\n# Parallelization\nNPAR=4 # change this to the number of nodes in the job" ("INCAR - Relaxation") "#For DOS Calcuations and to get the WAVECAR\n# I/O\nICHARG=1\nLWAVE=.TRUE.   #Write wavefunctions?\nLORBIT=11\nNEDOS=2000  # Number of DOS steps\n\n# Ionic\nIBRION=-1    #What type of calculation? \nISIF=2\nNSW=1\nLREAL=Auto\n\n# Electronic\nISMEAR=-5\nPREC=High\nALGO=Fast\nISPIN=1     # Electron spin, 1=nope, 2=account for spin\nNELM=100\nNELMIN=5\nEDIFF=1E-06  #energy difference to stop relaxation at\n\n# Parallelization\nNPAR=4 # change this to the number of nodes in the job"] -> w561
          tunnel: [w565 _ _ _ _ _ _ _] -> _
          frame "Read in from folder", Default {
            n345 = local read "Input Structure File"() -> (w569:path)
            n346 = Strip Path(path=w569) -> (stripped path=w568:path)  [unwired: 1 out]
            n347 = Build Path(base path=w568, name or relative path="INCAR") -> (appended path=w566:path)
            n348 = Read from Text File(file (use dialog)=w566) -> (text=w563:string, error out=w565:errorcluster)  [unwired: 3 in, 2 out]
            n349 = Empty String/Path?(string/path=w563) -> (empty?=w564:bool)
            n350 = case shown="True" w564 {
              tunnel: w563 -> [w570 _]
              tunnel: [w570 w571] -> w562
              frame False {
              }
              frame True {
                w571 = "#For Relaxation\n# I/O\nICHARG=1\nLWAVE=.FALSE.  #Write wavefunctions?\nLORBIT=11\nNEDOS=2000     # Number of DOS steps\n\n# Ionic\nIBRION=2     #What type of calculation? \nISIF=2     #Stress tensor and degrees of freedom?\nNSW=199\nLREAL=Auto\nEDIFFG=1E-04\n\n# Electronic\nISMEAR=0\nSIGMA=0.05\nPREC=High\nALGO=Fast\nISPIN=1     # Electron spin, 1=nope, 2=account for spin\nNELM=100\nNELMIN=5\nEDIFF=1E-06    #energy difference to stop relaxation at\n\n# Parallelization\nNPAR=4     # change this to the number of nodes in the job\n"  # INCAR - Relaxation Fixed Vol
              }
            }
          }
          frame "Relaxation" {
            w572 = "#For Relaxation\n# I/O\nICHARG=1\nLWAVE=.FALSE.  #Write wavefunctions?\nLORBIT=11\nNEDOS=2000     # Number of DOS steps\n\n# Ionic\nIBRION=2     #What type of calculation? \nISIF=3     #Stress tensor and degrees of freedom?\nNSW=199\nLREAL=Auto\nEDIFFG=1E-04\n\n# Electronic\nISMEAR=0\nSIGMA=0.05\nPREC=High\nALGO=Fast\nISPIN=1     # Electron spin, 1=nope, 2=account for spin\nNELM=100\nNELMIN=5\nEDIFF=1E-06    #energy difference to stop relaxation at\n\n# Parallelization\nNPAR=4     # change this to the number of nodes in the job\n"  # INCAR - Relaxation
          }
          frame "Dielectric Tensor" {
            w573 = "#For Dielectric Tensor\n# I/O\nICHARG=1\nLWAVE=.FALSE.  #Write wavefunctions?\nLORBIT=11\nNEDOS=2000     # Number of DOS steps\n\n# Ionic\nIBRION=8     #For Dielectric, use symmetry\nISIF=2     #Fixed Volume\nNSW=1\nLREAL=Auto\nEDIFFG=1E-04\nLEPSILON = .TRUE. #Find dielectric tensor\n\n# Electronic\nISMEAR=-5\nSIGMA=0.05\nPREC=High\nALGO=Fast\nISPIN=1     # Electron spin, 1=nope, 2=account for spin\nNELM=100\nNELMIN=5\nEDIFF=1E-06    #energy difference to stop relaxation at\n\n# Parallelization\nNPAR=4     # change this to the number of nodes in the job\n"  # INCAR - Relaxation
          }
          frame "Relaxation - Fixed Volume" {
            w574 = "#For Relaxation at a fixed volume\n# I/O\nICHARG=1\nLWAVE=.FALSE.  #Write wavefunctions?\nLORBIT=11\nNEDOS=2000     # Number of DOS steps\n\n# Ionic\nIBRION=2     #What type of calculation? \nISIF=2     #Fixed Volume\nNSW=199\nLREAL=Auto\nEDIFFG=1E-04\n\n# Electronic\nISMEAR=0\nSIGMA=0.05\nPREC=High\nALGO=Fast\nISPIN=1     # Electron spin, 1=nope, 2=account for spin\nNELM=100\nNELMIN=5\nEDIFF=1E-06    #energy difference to stop relaxation at\n\n# Parallelization\nNPAR=4     # change this to the number of nodes in the job\n"  # INCAR - Relaxation
          }
          frame "Nudged Elastic Band" {
            w575 = "#For Nudged Elastic Band Calculations\n# I/O\nICHARG=1\nLWAVE=.FALSE.  #Write wavefunctions?\nLORBIT=11\n\nICHAIN=0 # Tell TST VASP to do NEB\nLCLIMB=.TRUE.         # Climbing Image NEB\nIMAGES=5\nLGLOBAL=.TRUE. # Optimize NEB globally, not line by line\n\n# Ionic\nISIF=2 # fixed Volume\nNSW=399\nIOPT=1                # LBFGS optimizer\nIBRION=3              # Tell VASP to use TST optimizer\nPOTIM=0               # Tell VASP to use TST optimizer\nILBFGSMEM=20          # number of steps stored in LBFGS memory\nFDSTEP=5E-3           # Finite difference step size for line optimizer\nINVCURV=0.01          # Initial inverse curvature used to construct \nLBFGS Hessian\nMAXMOVE=0.2           # Maximum allowed step size\nLLINEOPT=.FALSE.      # Use a force based line minimizer for translation\nEDIFFG=-0.05          # break for ionic loop \n\n# Electronic\nISMEAR=0\nSIGMA=0.05\nPREC=High\nALGO=Fast\nISPIN=1     # Electron spin, 1=nope, 2=account for spin\nNELM=100\nNELMIN=5\nEDIFF=1E-06    #energy difference to stop relaxation at\n\n# Parallelization\nNPAR=4     # change this to the number of nodes in the job\n"  # INCAR - Relaxation
          }
          frame "DOS Only" {
          }
          frame "PARCHG" {
          }
          frame "DOS+WAVE" {
          }
        }
        n351 = local write "INCAR File"(w561) -> ()
      }
      event "Command": Value Change {
        n352 = event-data() -> ("NewVal"=w579:string)  [unwired: 1 in, 4 out]
        n353 = case shown="\"IDIPOL\"" w579 {
          tunnel: [_ "This flag determines how to construct the 'initial' charge density" "Write Wavefunctions?" "Write the local potential file? " "Write PROCAR or PROOUT?" "Number of DOS gridpoints (integer)" "How should ions be moved?" "Monopole, dipole and quadrupole corrections" "Degrees of freedom and stress tensor settings" "Dielectric Tensor Calculation.\nMake sure to set IBRION = -1, 7 or 8!" "Symmetry used in calculations" "Number of ionic steps (integer)" "Projection operators: Real or reciprocal space?" "When is ionic relaxation done? (real number).\nNegative numbers check forces, positive checks energy." "How are partial orrupancies set for each orbital?\nPairs with SIGMA. Can be a positive integer" "What is the smearing width in eV? (Real)" "What precision?" "Which electronic minimization algorithm?" "Spin polarization?" "Energy cutoff for the plane wave basis (PAW) set.\n|G+k| < Gcut, Encut = h/2m Gcut²" "Maximum number of electronic steps? (Integer)" "Minimum number of electronic steps? (Integer)" "When is electronic relaxation done? (real number).\nIn most cases the convergence speed is exponential." "How many bands are calculated in parallel?\nRecommend NPAR = sqrt(number of cores)" w637] -> w582
          tunnel: [_ string[] ["0  #From initial wave functions", "1  #Read from CHGCAR, and extrapolate ", "2  #Take superposition of atomic charge densities"] string[] [".FALSE.  #Don't write WAVECAR", ".TRUE.  #Write huge WAVECAR file"] string[] [".FALSE.  #Don't write LOCPOT", ".TRUE.  #Write LOCPOT"] string[] ["0  #Need WRIGS, write DOSCAR and PROCAR", "1  #Need WRIGS, write DOSCAR and lm-decomp PROCAR", "2  #Need WRIGS, write DOSCAR and lm-decomp PROCAR + phase", "5  #Need WRIGS, write DOSCAR and PROOUT", "10  #Write DOSCAR and PROCAR", "11  #Write DOSCAR and lm-decomp PROCAR", "12  #Write DOSCAR and lm-decomp PROCAR +phase"] string[] ["500  #Cheap and fast", "2000  #Standard", "5000  #You must be crazy"] string[] ["-1  #Don't move atoms", "0  #Molecular dynamics", "1  #Ionic relaxation quasi-newton (RMM-DIIS)", "2  #Ionic relaxation by conjugate gradient", "3  #Need SMASS, Ionic relaxation by damped molecular dynamics", "5  #Get Hessian and vibrational freqs, no symmetry", "6  #Get Hessian and vibrational freqs, use symmetry", "7  #Get Hessian and phonons by perturbation, no symmetry", "8  #Get Hessian and phonons by perturbation, use symmetry", "44  #Improved Dimer Method"] string[] ["1 #Correct along a", "2 #Correct along b", "3 #Correct along c", "4 #Correct all and display"] string[] ["0  # Stress tensor = no | relax ion = Yes | change cell = no | change vol = no", "1  # Stress tensor = Trace | relax ion = Yes | change cell = no | change vol = no", "2  # Stress tensor = Yes | relax ion = Yes | change cell = no | change vol = no", "3  # Stress tensor = Yes | relax ion = Yes | change cell = Yes | change vol = yes", "4  # Stress tensor = Yes | relax ion = Yes | change cell = Yes | change vol = no", "5  # Stress tensor = Yes | relax ion = no | change cell = Yes | change vol = no", "6  # Stress tensor = Yes | relax ion = no | change cell = Yes | change vol = yes", "7  # Stress tensor = Yes | relax ion = no | change cell = no | change vol = yes"] string[] [".TRUE. #Calculate Dielectric Tensor", ".FALSE. # No dielectric tensor"] string[] ["-1 #No Symmetry", "0 #No Symmetry", "1 #Symmetry for PseudoPots", "2 #Symmetry for PAW", "3 #Symmetry only for forces/stress"] string[] ["50  #Fast", "199  #Standard", "500  #Very long"] string[] [".TRUE.  # real space proj", ".FALSE.  #reciprocal space proj", "On  # real space optimized proj", "Auto  # real space, fully auto optimized proj"] string[] ["1E-4  # Rough calculation", "1E-6  #Standard", "1E-8  #Very accurate"] string[] ["-5  #Tetrahedron with Blochl corrections (0 centered)", "-4  #Tetrahedron method, 0 centered", "-3  #Smearing loop with SMEARINGS tag", "-2  #Read from WAVECAR, FERWE and FERDO", "-1  #Fermi smearing", "0  #Guassian Smearing", "1  #Methfessal-Paxton order 1"] string[] ["0.2  #default", "0.05  #standard"] string[] ["Low", "Medium", "High  #standard", "Normal  #recommended", "Single", "Accurate"] string[] ["Normal  #Davidson scheme", "Fast  #Mixture between Davidson and RMM-DIIS", "VeryFast  #RMM-DIIS", "Conjugate  #All band update using conjugate gradient", "Damped  #Dampled velocity friction", "Subrot  #Subspace rotation by orbitals", "Eigenval  #Read from WAVECAR", "None  #1-electron energies, read from WAVECAR", "CHI  #Response functions only", "GW0  #Single shot G0W0 calculations, G is updated", "GW  #Single shot G0W0 calculations, G and W is updated", "scGW0  #self-consistent GW calculations using off-diagonal, G updated", "scGW  #self-consistent GW calculations using off-diagonal, G and W updated"] string[] ["1  #non-spin polarized calc", "2  #electrons have spin!"] string[] ["274.342 # Cd Standard", "500 # Very High"] string[] ["40  #Recommended", "60  #Default", "100  #Standard"] string[] ["2  #Default", "5  #Standard"] string[] ["1E-4  #Default", "1E-6  #Standard"] string[] ["2  #Default", "4  #Standard", "8  #Tough calculation"] w629] -> w581
          frame Default {
          }
          frame "ICHARG" {
          }
          frame "LWAVE" {
          }
          frame "LVTOT" {
          }
          frame "LORBIT" {
          }
          frame "NEDOS" {
          }
          frame "IBRION" {
          }
          frame "IDIPOL" {
          }
          frame "ISIF" {
          }
          frame "LEPSILON" {
          }
          frame "ISYM" {
          }
          frame "NSW" {
          }
          frame "LREAL" {
          }
          frame "EDIFFG" {
          }
          frame "ISMEAR" {
          }
          frame "SIGMA" {
          }
          frame "PREC" {
          }
          frame "ALGO" {
          }
          frame "ISPIN" {
          }
          frame "ENCUT" {
          }
          frame "NELM" {
          }
          frame "NELMIN" {
          }
          frame "EDIFF" {
          }
          frame "NPAR" {
          }
          frame "NELECT" {
            w637 = "How many electrons?\nDefault level is Cd*12 + Te*6"  # How many electrons? Default level is Cd*12 + Te*6
            n354 = local read "Current Atomic Structure"() -> (w636:T3)
            n355 = Unbundle By Name(w636) -> ("Atoms Array"=w635:T20)
            n356 = for {
              tunnel: w635 -> [w645] mode=indexing
              tunnel: [w640] -> w634 mode=indexing
              n357 = Unbundle By Name(w645) -> ("Atom Name"=w639:string, "Positions (Direct)"=w644:dbl[][])
              n358 = case shown="Default" w639 {
                tunnel: [6 ("x") 1 ("x") 12 ("x")] -> w638
                frame "#Te", "Te" {
                }
                frame Default {
                }
                frame "#Cd", "Cd" {
                }
              }
              n359 = Index Array(array=w644, index (col)=0 ("disabled index (col)")) -> (element=w642:dbl[])  [unwired: 1 in]
              n360 = Array Size(array=w642) -> (size(s)=w641:i32)
              n361 = Multiply(x=w638, y=w641) -> (x*y=w640:i32)
            }
            n362 = Add Array Elements(numeric array=w634) -> (sum=w633:i32)
            n363 = Number To Decimal String(number=w633) -> (decimal integer string=w632:string)  [unwired: 1 in]
            n364 = Concatenate Strings(w632, "  #Default Cd*12+Te*6" ("string")) -> (w630:string)
            n365 = Build Array(w630) -> (w629:string[])
          }
        }
        "Description" <- w582
        n366 = Index Array(array=w581) -> (element=w580:string)  [unwired: 1 in]
        n367 = property on="Value" class="CmbBox"("Value"=w580, "Strings[]"=w581) -> ()  [unwired: 2 in, 2 out]
      }
      event "INCAR File": Shortcut Menu Activation? {
        n368 = event-data() -> ("MenuRef"=w650:refnum<k9>)  [unwired: 1 in, 5 out]
        n369 = Insert Menu Items(8:string[] ["---", "Add line here", "Add to end"] ("item names"), 9:w650) -> ()  [unwired: 4 in, 3 out]
        n370 = event-data() -> ()  [unwired: 2 in, 1 out]
      }
      event "INCAR File": Shortcut Menu Selection (User) {
        n371 = event-data() -> ("ItemTag"=w653:string, "Coords"=w652:T24)  [unwired: 1 in, 5 out]
        n372 = case shown="True" "Write # comment" {
          tunnel: "Value" -> [w672 w673]
          tunnel: [w670 w673] -> w655
          frame False {
            n373 = Search/Split String(string=w672, search string/char (-)="#") -> (substring before match=w670:string)  [unwired: 1 in, 2 out]
          }
          frame True {
          }
        }
        n374 = Concatenate Strings("\n", "Command", "=" ("string"), w655) -> (w654:string)
        n375 = case shown="\"Add line here\"" w653 {
          tunnel: w654 -> [_ w660 w666]
          tunnel: w652 -> [_ _ w669]
          frame Default {
          }
          frame "Add to end" {
            n376 = local read "INCAR File"() -> (w662:string)
            n377 = Concatenate Strings(w662, w660) -> (w661:string)
            n378 = local write "INCAR File"(w661) -> ()
          }
          frame "Add line here" {
            n379 = invoke on="INCAR File" class="Str" method="ByteOffFromPt"("Point"=w669) -> ("ByteOffFromPt"=w668:i32)  [unwired: 3 in, 3 out]
